vi "WK6425_Tests.vi"(8 "error in (no error)":errorcluster, 11 "WK6425 in":refnum<class "WK6425.lvclass">) -> (0 "error out":errorcluster, 3 "WK6425 out":refnum<class "WK6425.lvclass">)   [LabVIEW 2018, in "WK6425.lvclass"]
uses:
  WK6425.lvclass
  <vilib>/Platform/TimedLoop/XDataNode/timing_clust.ctl
  <vilib>/Platform/TimedLoop/XDataNode/nitl_modes.ctl
  <vilib>/Platform/TimedLoop/XDataNode/wakeup.ctl
  InstrumentSetup.vi
  <vilib>/platform/TimedLoop/XDataNode/XDataNode.xnode
  <vilib>/Platform/TimedLoop/XDataNode/XDNodeRunTimeDep.lvlib
  InstrControl.lvclass
panel:
  out "Capacitance in pF":dbl
  out "Resistance in MOhm":dbl
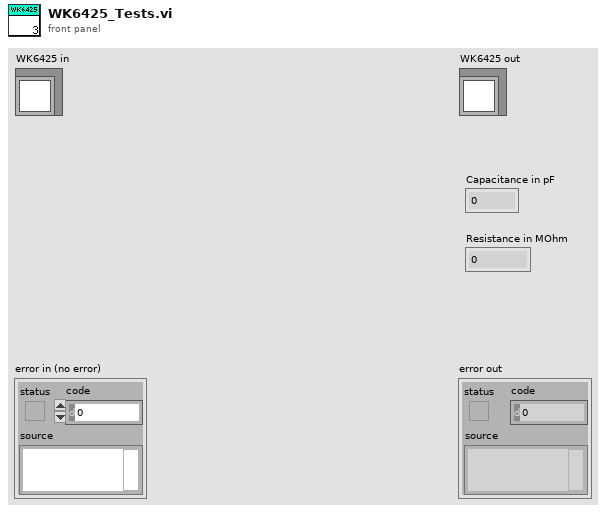
[diagram p1: front panel]
types:
  T1 = cluster{"KE 2410":cluster{"Instrument name":string, "GPIB address":string, "Instrument type":u16}, "KE 6517":cluster{"Instrument name":string, "GPIB address":string, "Instrument type":u16}, "KE 487":cluster{"Instrument name":string, "GPIB address":string, "Instrument type":u16}, "KE 487_2":cluster{"Instrument name":string, "GPIB address":string, "Instrument type":u16}, "KE 236":cluster{"Instrument name":string, "GPIB address":string, "Instrument type":u16}, "WK 6440B":cluster{"Instrument name":string, "GPIB address":string, "Instrument type":u16}, "WK 6425":cluster{"Instrument name":string, "GPIB address":string, "Instrument type":u16}, "Pickering Matrix":cluster{"Instrument name":string, "GPIB address":string, "Instrument type":u16}, "KE 2000":cluster{"Instrument name":string, "GPIB address":string, "Instrument type":u16}, "KE 2657A":cluster{"Instrument name":string, "GPIB address":string, "Instrument type":u16}, "Prague Pickering Matrix":cluster{"Instrument name":string, "GPIB address":string, "Instrument type":u16}}
  T2 = cluster{"RC Configuration":u16, "AC amplitude [V]":dbl, "AC frequency [Hz]":i32, "WK6425":refnum<class "WK6425.lvclass">}
  T3 = typedef "XDNodeRunTimeDep.lvlib/timing_clust.ctl" = cluster{"Expected End [f-1]":u64, "Actual End [f-1]":u64, "Finished Late? [f-1]":bool, "Expected End [i-1]":u64, "Actual End [i-1]":u64, "Finished Late? [i-1]":bool, "Expected Start [i]":u64, "Actual Start [i]":u64, "Expected Start [f]":u64, "Actual Start [f]":u64, "Source Name":string, "Structure Name":string, "Period":i64, "Deadline":i64, "Offset":i64, "Start":i64, "Priority":i32, "Timeout":i32, "Mode":T4, "Wakeup Reason":T5, "Error":errorcluster, "Source Type":string, "Secondary Source Type":string, "Global End Time":u64, "Global Start Time":u64, "Frame Duration":u64, "Iteration Duration":u64, "Assigned CPU":i32, "I/O Scan Engine Mode":u32}
  T4 = typedef "XDNodeRunTimeDep.lvlib/nitl_modes.ctl" = enum32{"No Change", "Process missed periods, maintain original phase", "Discard missed periods, maintain original phase", "Process missed periods, ignore original phase", "Discard missed periods, ignore original phase"}
  T5 = typedef "XDNodeRunTimeDep.lvlib/wakeup.ctl" = enum32{"Normal", "Aborted", "Asynchronous wakeup", "Timing source error", "Timed loop error", "Timeout"}
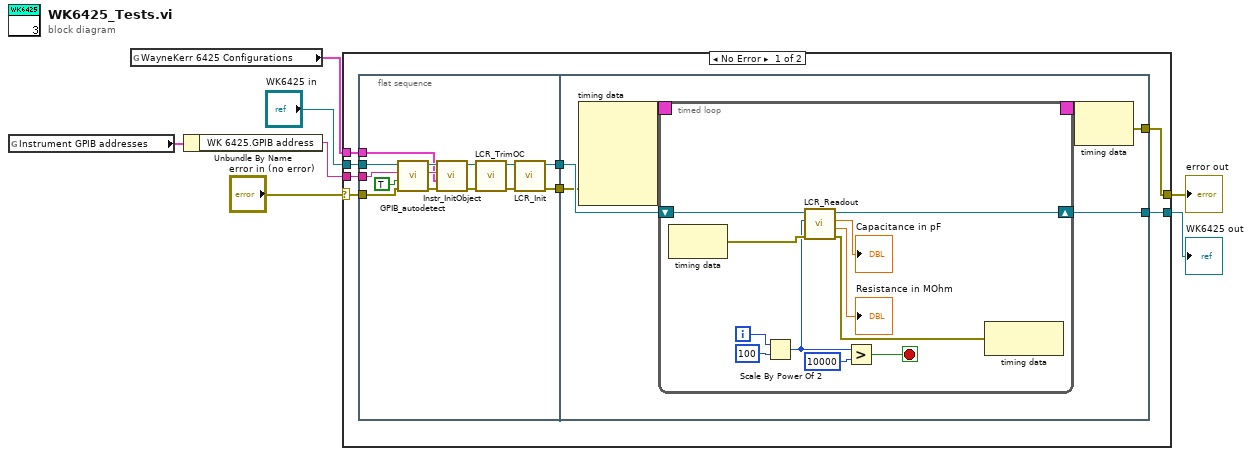
[diagram p0: block diagram]
diagram:
  n1 = global read "InstrumentSetup.vi" "Instrument GPIB addresses"() -> (w3:T1)
  n2 = global read "InstrumentSetup.vi" "WayneKerr 6425 Configurations"() -> (w1:T2)
  n3 = Unbundle By Name(w3) -> ("WK 6425.GPIB address"=w2:string)
  n4 = case shown="No Error" "error in (no error)" {
    selector: "error in (no error)" -> [w14 w58]
    tunnel: [w12 w58] -> w6
    tunnel: [w13 w57] -> w4
    tunnel: "WK6425 in" -> [w15 w57]
    tunnel: w2 -> [w9 _]
    tunnel: w1 -> [w8 _]
    frame No Error {
      n5 = flat-sequence {
        tunnel: w15 -> [w22]
        tunnel: w14 -> [w19]
        tunnel: [w29] -> w11
        tunnel: [w28] -> w10
        tunnel: w9 -> [w18]
        tunnel: w8 -> [w17]
        tunnel: w11 -> [w32]
        tunnel: w10 -> [w30]
        tunnel: [w33] -> w12
        tunnel: [w31] -> w13
        frame #0 {
          n6 = call-dynamic "GPIB_autodetect.vi"("error in (no error)"=w19, "Verify GPIB address"=TRUE, "Instrument GPIB address in"=w18, "InstrControl in"=w22) -> ("error out"=w25:errorcluster, "Instrument GPIB address"=w23:string, "InstrControl out"=w24:refnum<class "WK6425.lvclass">)  [unwired: 5 in]
          n7 = call-dynamic "Instr_InitObject.vi"("error in (no error)"=w25, "Instrument Configuration"=w17, "GPIB Address"=w23, "WK6425 in"=w24) -> ("error out"=w20:errorcluster, "WK6425 out"=w21:refnum<class "WK6425.lvclass">)  [unwired: 6 in]
          n8 = call-dynamic "LCR_TrimOC.vi"("error in (no error)"=w20, "LCRControl in"=w21) -> ("error out"=w26:errorcluster, "LCRControl out"=w27:refnum<class "WK6425.lvclass">)  [unwired: 8 in]
          n9 = call-dynamic "LCR_Init.vi"("error in (no error)"=w26, "LCRControl in"=w27) -> ("error out"=w28:errorcluster, "LCRControl out"=w29:refnum<class "WK6425.lvclass">)  [unwired: 8 in]
        }
        frame #1 {
          n10 = node-c288(w30) -> (w35:T3)  [unwired: 4 in]
          n11 = timed-loop {
            timing: w35 -> [_]
            timing-out: [_] -> w34
            shift-right: [w39] -> w31
            shift-left: w32 -> [w36]
            i -> [w41]
            stop <- w43 stop-if-true
            n12 = node-c288() -> (w46:errorcluster)  [unwired: 1 in]
            n13 = Scale By Power Of 2(n=w41, x=100) -> (x*2^n=w40:i32)
            n14 = call-dynamic "LCR_Readout.vi"("error in (no error)"=w46, "Frequency in Hz"=w40, "WK6425 in"=w36) -> ("error out"=w45:errorcluster, "Resistance in Ohm"=→"Resistance in MOhm":dbl, "Capacitance in pF"=→"Capacitance in pF":dbl, "WK6425 out"=w39:refnum<class "WK6425.lvclass">)  [unwired: 5 in]
            n15 = Greater?(x=w40, y=10000) -> (0:w43:bool)
            n16 = node-c288(w45) -> ()  [unwired: 1 out]
          }
          n17 = node-c288(w34) -> (w33:errorcluster)
        }
      }
    }
    frame Error {
    }
  }
  "error out" <- w6
  "WK6425 out" <- w4
